vi "MicroPulse - decode error log report.vi"(9 "data":u8[](array[numeric]), 11 "No. of Logs":u16) -> (1 "error report":string)   [LabVIEW 2026, in "MicroPulse_Driver.lvlib"]
uses:
  MicroPulse_Driver.lvlib
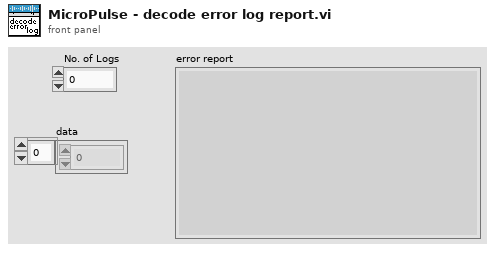
[diagram p1: front panel]
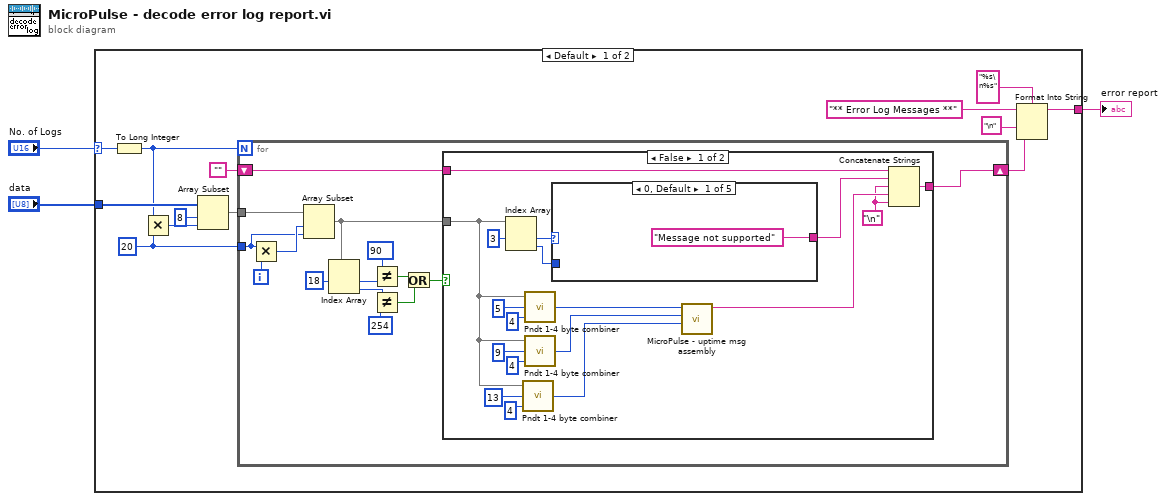
[diagram p0: block diagram]
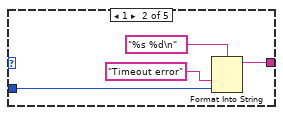
[diagram p2: hidden frame]
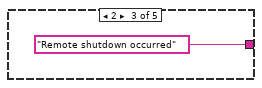
[diagram p3: hidden frame]
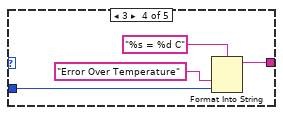
[diagram p4: hidden frame]
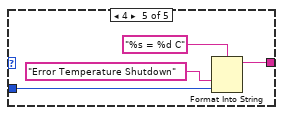
[diagram p5: hidden frame]
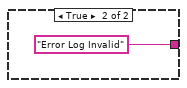
[diagram p6: hidden frame]
diagram:
  n1 = case shown="Default" "No. of Logs" {
    selector: "No. of Logs" -> [w4 _]
    tunnel: [w9 _] -> w3
    tunnel: "data" -> [w8 _]
    frame Default {
      w5 = 20
      n2 = To Long Integer(number=w4) -> (32bit integer=w6:i32)
      n3 = Multiply(x=w6, y=w5) -> (x*y=w7:i32)
      n4 = Array Subset(array=w8, index=8 ("y"), length=w7) -> (w16:u8[])
      n5 = for {
        N: w6 -> [_]
        tunnel: w16 -> [w31]
        shift-right: [w27] -> w10
        shift-left: "" -> [w28]
        tunnel: w5 -> [w17]
        i -> [w30]
        n6 = Multiply(x=w17, y=w30) -> (x*y=w29:i32)
        n7 = Array Subset(array=w31, index=w29, length=w17) -> (w26:u8[])
        n8 = Index Array(array=w26, index #1=18 ("x")) -> (element #1=w24:u8, element #2=w22:u8)  [unwired: 1 in]
        n9 = Not Equal?(x=u8 90, y=w24) -> (x != y?=w20:bool)
        n10 = Not Equal?(x=w22, y=u8 254 ("x")) -> (x != y?=w19:bool)
        n11 = Or(x=w20, y=w19) -> (x .or. y?=w18:bool)
        n12 = case shown="False" w18 {
          tunnel: w28 -> [w46 _]
          tunnel: [w45 "Error Log Invalid"] -> w27
          tunnel: w26 -> [w34 _]
          frame False {
            w32 = "\n"
            n13 = Index Array(array=w34, index #1=3 ("index")) -> (element #1=w48:u8, element #2=w47:u8)  [unwired: 1 in]
            n14 = call "Pndt 1-4 byte combiner.vi"("#bytes"=4 ("index"), "start index [0]"=13 ("index"), "[U8] count bytes"=w34) -> ("U32"=w35:u32)
            n15 = call "Pndt 1-4 byte combiner.vi"("#bytes"=4 ("index"), "start index [0]"=5 ("index"), "[U8] count bytes"=w34) -> ("U32"=w41:u32)
            n16 = call "Pndt 1-4 byte combiner.vi"("#bytes"=4 ("index"), "start index [0]"=9 ("index"), "[U8] count bytes"=w34) -> ("U32"=w40:u32)
            n17 = case shown="0, Default" w48 {
              tunnel: ["Message not supported" w51 "Remote shutdown occurred" w56 w60] -> w44
              tunnel: w47 -> [_ w52 _ w57 w61]
              frame 0, Default {
              }
              frame 1 {
                n18 = Format Into String(format string="%s %d\n", "Timeout error", w52) -> (resulting string=w51:string)  [unwired: 2 in, 1 out]
              }
              frame 2 {
              }
              frame 3 {
                n19 = Format Into String(format string="%s = %d C", "Error Over Temperature", w57) -> (resulting string=w56:string)  [unwired: 2 in, 1 out]
              }
              frame 4 {
                n20 = Format Into String(format string="%s = %d C", "Error Temperature Shutdown", w61) -> (resulting string=w60:string)  [unwired: 2 in, 1 out]
              }
            }
            n21 = call "MicroPulse - uptime msg assembly.vi"("SRST"=w35, "RST"=w40, "Uptime"=w41) -> ("String"=w33:string)  [unwired: 8 in]
            n22 = Concatenate Strings(w46, w44, w32, w33, w32) -> (w45:string)
          }
          frame True {
          }
        }
      }
      n23 = Format Into String(format string="%s\n%s", initial string="** Error Log Messages **", "\n" ("input 1"), w10) -> (resulting string=w9:string)  [unwired: 1 in, 1 out]
    }
    frame 0 {
    }
  }
  "error report" <- w3
